vi "Get Item Type.vi"(8 "error in (no error)":errorcluster, 11 "ClickableText in":refnum<class "ClickableText.lvclass">) -> (0 "error out":errorcluster, 2 "DNL_Type":T1=enum."New VI", 3 "ClickableText out":refnum<class "ClickableText.lvclass">)   [LabVIEW 2009, in "NavScreen.lvlib" / "ClickableText.lvclass"]
uses:
  ClickableText.lvclass
  ItemData_Type.ctl
  ClickableText.lvclass/ClickableText.ctl
  NavScreen.lvlib
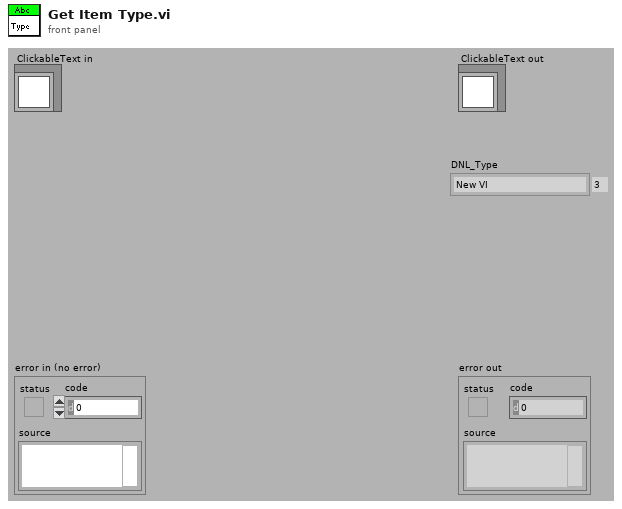
[diagram p1: front panel]
types:
  T1 = typedef "NavScreen.lvlib/ItemData_Type.ctl" = enum16{"None", "Folder", "New Project", "New VI", "Find", "VI", "Project", "New from template", "RT Project Wizard", "PDA Project Wizard", "Control", "Library", "Class", "XControl", "Runtime menu"}
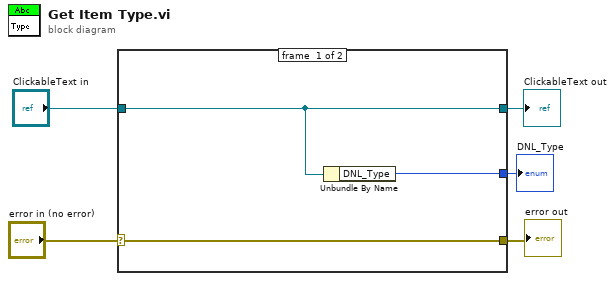
[diagram p0: block diagram]
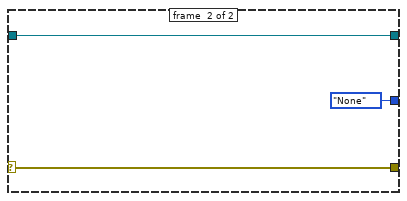
[diagram p2: hidden frame]
diagram:
  n1 = case shown="No Error" "error in (no error)" {
    selector: "error in (no error)" -> [w8 w11]
    tunnel: [w8 w11] -> w4
    tunnel: [w7 w10] -> w2
    tunnel: "ClickableText in" -> [w7 w10]
    tunnel: [w6 ItemData_Type."None" ("DNL_Type")] -> w1
    frame #0 {
      n2 = Unbundle By Name(w7) -> ("DNL_Type"=w6:T1)
    }
    frame #1 {
    }
  }
  "error out" <- w4
  "ClickableText out" <- w2
  "DNL_Type" <- w1
